vi "BB2014Beta_WPI_DashboardPanel Resized.vi"(6 "Sizing Refnums":T2, 8 "error in (no error)":errorcluster, 9 "Origin":cluster{"H":i16, "V":i16}, 10 "NewBnds":T1, 11 "Size Constraints":cluster{"min tab width":i32, "w/h":dbl}) -> (0 "error out":errorcluster)   [LabVIEW 2014]
uses:
  <vilib>/Utility/miscctls.llb/LVRectTypeDef.ctl
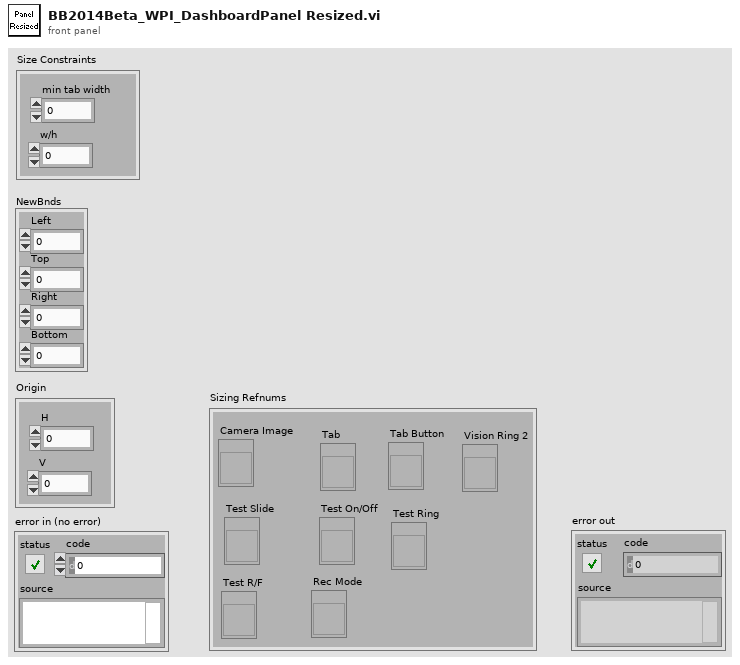
[diagram p1: front panel]
types:
  T1 = typedef "LVRectTypeDef.ctl" = cluster{"Left":i16, "Top":i16, "Right":i16, "Bottom":i16}
  T2 = cluster{"Camera Image":refnum<vi>, "Tab":refnum<vi>, "Tab Button":refnum<vi>, "Vision Ring 2":refnum<vi>, "Test Slide":refnum<vi>, "Test On/Off":refnum<vi>, "Test Ring":refnum<vi>, "Test R/F":refnum<vi>, "Rec Mode":refnum<vi>}
  T3 = typedef "LVPositionTypeDef.ctl" = cluster{"Left":i32, "Top":i32}
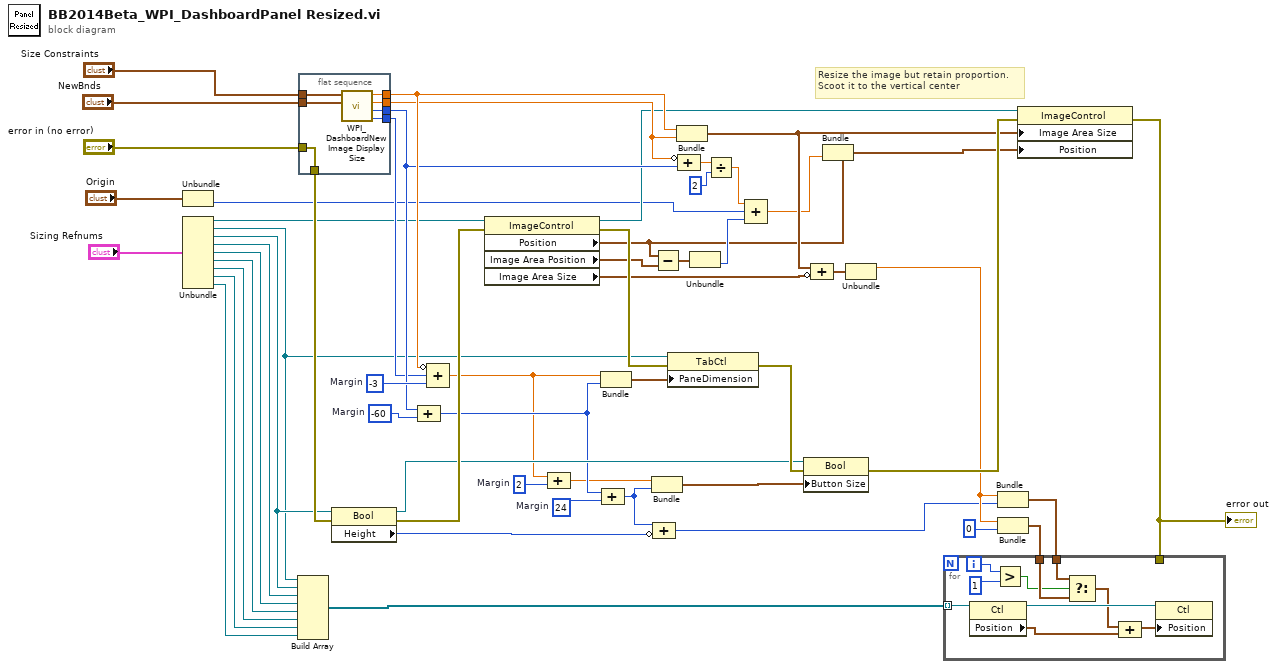
[diagram p0: block diagram]
diagram:
  w34 = 24  # Margin
  w32 = 2  # Margin
  w28 = -60  # Margin
  w38 = -3  # Margin
  # "Resize the image but retain proportion.\nScoot it to the vertical center"
  n1 = Unbundle("Origin") -> ("V"=w7:i16)  [unwired: 1 out]
  n2 = Unbundle("Sizing Refnums") -> ("Camera Image"=w1:refnum<vi>, "Tab"=w2:refnum<vi>, "Tab Button"=w10:refnum<vi>, "Vision Ring 2"=w51:refnum<vi>, "Test Slide"=w52:refnum<vi>, "Test On/Off"=w53:refnum<vi>, "Test Ring"=w54:refnum<vi>, "Test R/F"=w55:refnum<vi>, "Rec Mode"=w56:refnum<vi>)
  n3 = Build Array(w2, w10, w51, w52, w53, w54, w55, w56) -> (w50:refnum<vi>[])
  n4 = flat-sequence {
    tunnel: "NewBnds" -> [w63]
    tunnel: "Size Constraints" -> [w62]
    tunnel: [w61] -> w26
    tunnel: [w60] -> w35
    tunnel: [w59] -> w36
    tunnel: [w58] -> w37
    tunnel: [w57] -> w49
    tunnel: "error in (no error)" -> [w57]
    frame #0 {
      n5 = call <vilib>:"WPI_DashboardNew Image Display Size.vi"("NewBnds"=w63, "Size Constraints"=w62) -> ("Window Width"=w61:i16, "Window Height"=w59:i16, "Height"=w60:dbl, "Width"=w58:dbl)  [unwired: 6 in]
    }
  }
  n6 = property class="Bool"(reference=w10, error in=w49) -> (reference out=w42:refnum<vi>, error out=w48:errorcluster, "Height"=w40:u32)
  n7 = Compound Arithmetic op=unknown(w36, w28) -> (w33:i32)
  n8 = Compound Arithmetic op=ADD(invert w37, w26, w38) -> (w31:dbl)
  n9 = property class="ImageControl"(reference=w1, error in=w48) -> (reference out=w19:refnum<vi>, error out=w45:errorcluster, "Position"=w18:T3, "Image Area Position"=w13:cluster{"Left":i32, "Top":i32}, "Image Area Size"=w24:cluster{"Width":u32, "Height":u32})
  n10 = Compound Arithmetic op=ADD(w31, w32) -> (w30:dbl)
  n11 = Bundle(w31, w33) -> (w27:cluster{dbl, i32})  [unwired: 1 in]
  n12 = Compound Arithmetic op=ADD(w33, w34) -> (w39:i32)
  n13 = Bundle(w30, w39) -> (w29:cluster{dbl, i32})  [unwired: 1 in]
  n14 = Subtract(x=w18, y=w13) -> (x-y=w20:T3)
  n15 = Compound Arithmetic op=ADD(w39, invert w40) -> (w41:u32)
  n16 = property class="TabCtl"(reference=w2, error in=w45, "PaneDimension"=w27) -> (error out=w46:errorcluster)  [unwired: 1 out]
  n17 = Bundle("Width"=w37, "Height"=w35) -> (w22:cluster{"Width":dbl, "Height":dbl})  [unwired: 1 in]
  n18 = Compound Arithmetic op=ADD(invert w35, w36) -> (w14:dbl)
  n19 = Unbundle(w20) -> ("Top"=w21:i32)  [unwired: 1 out]
  n20 = Divide(x=w14, y=2) -> (x/y=w16:dbl)
  n21 = Compound Arithmetic op=ADD(w16, w7, w21) -> (w17:dbl)
  n22 = property class="Bool"(reference=w42, error in=w46, "Button Size"=w29) -> (error out=w47:errorcluster)  [unwired: 1 out]
  n23 = Compound Arithmetic op=ADD(w22, invert w24) -> (w25:cluster{"Width":dbl, "Height":dbl})
  n24 = Bundle(cluster=w18, "Top"=w17) -> (w23:T3)  [unwired: 1 in]
  n25 = Unbundle(w25) -> ("Width"=w43:dbl)  [unwired: 1 out]
  n26 = Bundle("Width"=w43, w41) -> (w12:cluster{"Width":dbl, u32})  [unwired: 1 in]
  n27 = Bundle("Width"=w43, 0) -> (w11:cluster{"Width":dbl, i32})  [unwired: 1 in]
  n28 = property class="ImageControl"(reference=w19, error in=w47, "Image Area Size"=w22, "Position"=w23) -> (error out=w6:errorcluster)  [unwired: 1 out]
  "error out" <- w6
  n29 = for {
    tunnel: w50 -> [w73] mode=indexing
    tunnel: w12 -> [w68]
    tunnel: w11 -> [w67]
    tunnel: w6 -> [_]
    i -> [w66]
    n30 = property class="Ctl"(reference=w73) -> (reference out=w72:refnum<vi>, "Position"=w71:T3)  [unwired: 1 in, 1 out]
    n31 = Greater?(x=w66, y=1) -> (0:w64:bool)
    n32 = Select(t=w68, s=w64, f=w67) -> (s? t:f=w69:cluster{"Width":dbl, u32})
    n33 = Compound Arithmetic op=ADD(w69, w71) -> (w70:cluster{dbl, u32})
    n34 = property class="Ctl"(reference=w72, "Position"=w70) -> ()  [unwired: 1 in, 2 out]
  }
